vi "Response.vi"(8 "error in (no error)":errorcluster, 11 "Node Ptr":T2 format="%.0x") -> (0 "error out":errorcluster)   [LabVIEW 2018, in "Instrument Addon System Explorer.lvlib"]
uses:
  Instrument Addon System Explorer.lvlib
  <vilib>/NI Veristand/Custom Device API/Custom Device Item Ref.ctl
  Addon Shared/Types/Response Wait Type.ctl
  NationalInstruments.VeriStand.SystemStorageUI
  Addon Shared/Types/FG Control.ctl
  NationalInstruments.VeriStand.SystemStorage
  Addon Shared/SubVIs/Constants.vi
  <vilib>/NI Veristand/Custom Device API/NI VeriStand - Get Item Property.vi
  <vilib>/NI Veristand/Custom Device API/Get Item Property (String).vi
  <vilib>/NI Veristand/Custom Device API/Get Item Property (String Array).vi
  <vilib>/NI Veristand/Custom Device API/Get Item Property (Double).vi
  <vilib>/NI Veristand/Custom Device API/Get Item Property (U32).vi
  <vilib>/NI Veristand/Custom Device API/Get Item Property (Boolean).vi
  <vilib>/NI Veristand/Custom Device API/NI VeriStand - Set Item Property.vi
  <vilib>/NI Veristand/Custom Device API/Set Item Property (String).vi
  <vilib>/NI Veristand/Custom Device API/Set Item Property (String Array).vi
  <vilib>/NI Veristand/Custom Device API/Set Item Property (Double).vi
  <vilib>/NI Veristand/Custom Device API/Set Item Property (U32).vi
  <vilib>/NI Veristand/Custom Device API/Set Item Property (Boolean).vi
  <vilib>/NI Veristand/Custom Device API/Custom Device API.lvlib
  Addon Shared/Instrument Addon Shared.lvlib
  <vilib>/NI Veristand/UI Controls/Single Node Browser/NI_VS UI Single Node Browser.lvlib
panel:
  in  "Type Value U32":u32=100 caption="Byte Count Value"
  in  "Channel":refnum<k24>(container) caption="Value"
  in  "Use Channel?":bool
  in  "Linkages":i32(listbox)
  in  "MetaData":string(combo) caption="Available Data Channels"
  in  "Response":string caption="Response Format ( Use [] to define a variable )"
  in  "Header 2":cluster{"Section Name":string}={"Section Name"="Response Message Settings"}
  in  "Wait Type":T1
  in  "Type Value DBL":dbl=100.0 caption="Byte Count Value" format="%#_p"
  in  "SHDocVw.IWebBrowser":refnum<k7>(container)
  in  "Header":cluster{"Section Name":string}={"Section Name"="Response Settings"}
  in  "Description":string
  out "Name":string
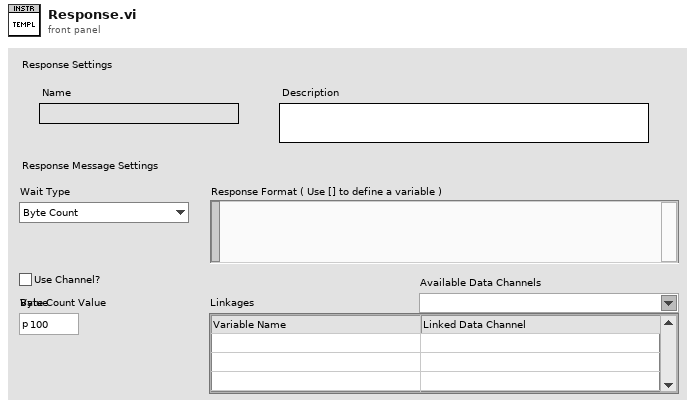
[diagram p1: front panel]
types:
  T1 = typedef "Instrument Addon Shared.lvlib/Response Wait Type.ctl" = enum16{"Byte Count", "Wait sec"}
  T2 = typedef "Custom Device API.lvlib/Custom Device Item Ref.ctl" = u64
  T3 = typedef "Instrument Addon Shared.lvlib/FG Control.ctl" = enum16{"Get", "Set"}
  T4 = typedef "Instrument Addon Shared.lvlib/Response Parameters.ctl" = cluster{"Response":string, "Linked Channels":T5[], "Type Value":dbl, "Wait Type":T1, "Use Channel":bool, "Channel Path":string}
  T5 = typedef "Instrument Addon Shared.lvlib/Linked Channel Cluster.ctl" = cluster{"Variable Name":string, "GUID":string}
  T6 = typedef "Custom Device API.lvlib/Custom Device Item Info.ctl" = cluster{"Name":string, "Is Channel":bool, "GUID":string, "Is Waveform":bool}
  T7 = typedef "Custom Device API.lvlib/Custom Device Commands.ctl" = enum16{"Default", "Item renamed", "Shutdown", "Dynamic button pressed"}
  T8 = typedef "NI_VS UI Single Node Browser.lvlib/Node Ref.ctl" = refnum<k24>
  T9 = typedef "Custom Device API.lvlib/Custom Device Pointer.ctl" = refnum<k24>
  T10 = typedef "LVComboBoxStrsAndValuesArrayTypeDef.ctl" = cluster{"String":string, "Value":string}[]
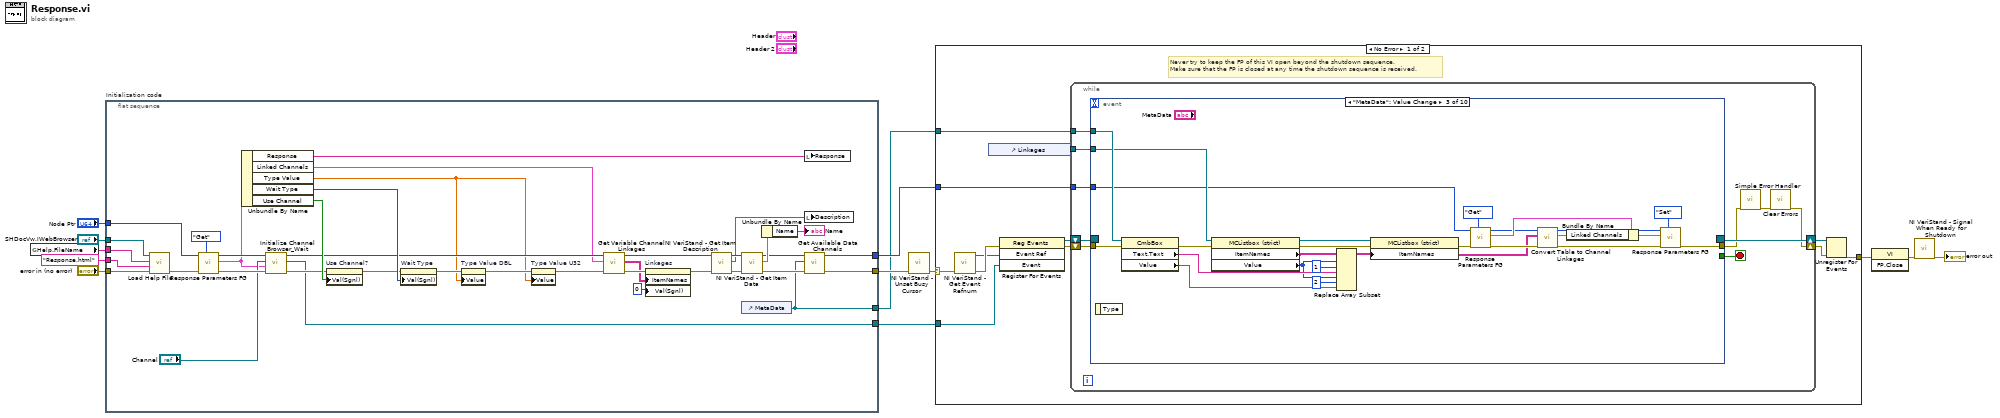
[diagram p0: block diagram]
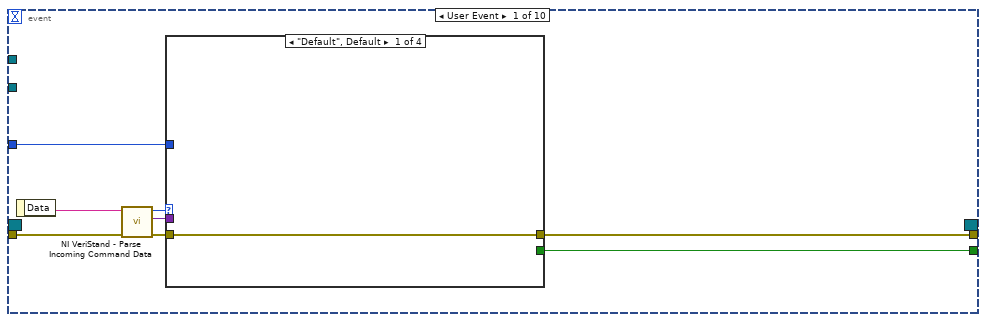
[diagram p2: hidden frame]
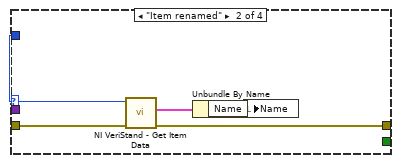
[diagram p3: hidden frame]
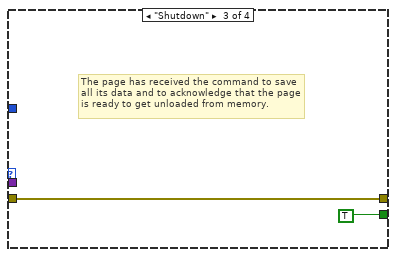
[diagram p4: hidden frame]
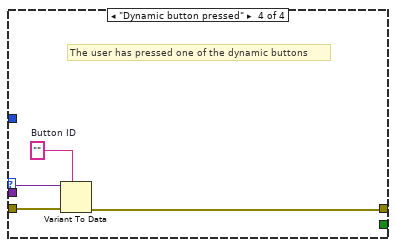
[diagram p5: hidden frame]
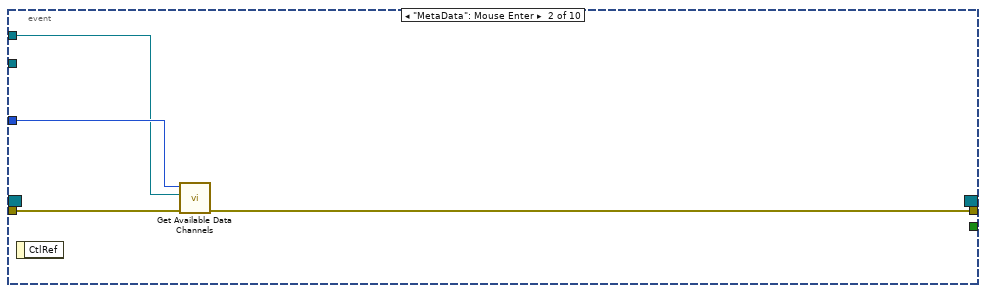
[diagram p6: hidden frame]
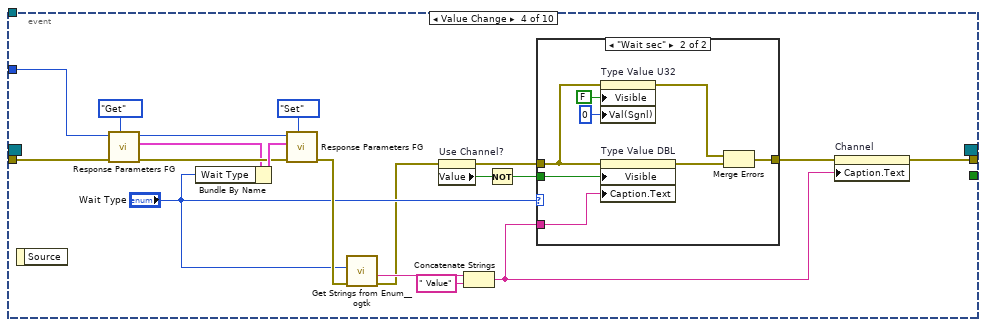
[diagram p7: hidden frame]
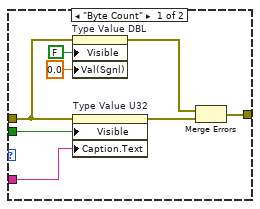
[diagram p8: hidden frame]
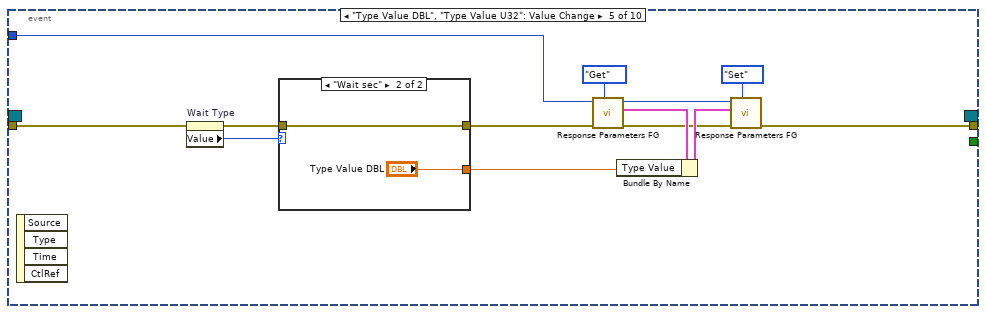
[diagram p9: hidden frame]
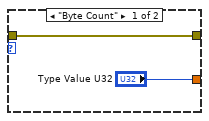
[diagram p10: hidden frame]
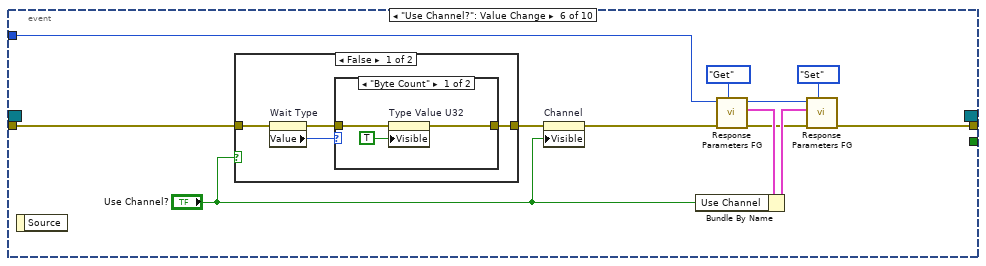
[diagram p11: hidden frame]
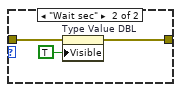
[diagram p12: hidden frame]
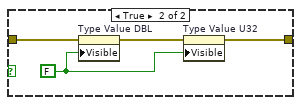
[diagram p13: hidden frame]
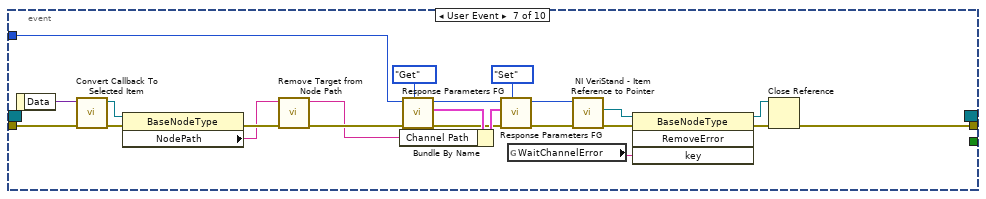
[diagram p14: hidden frame]
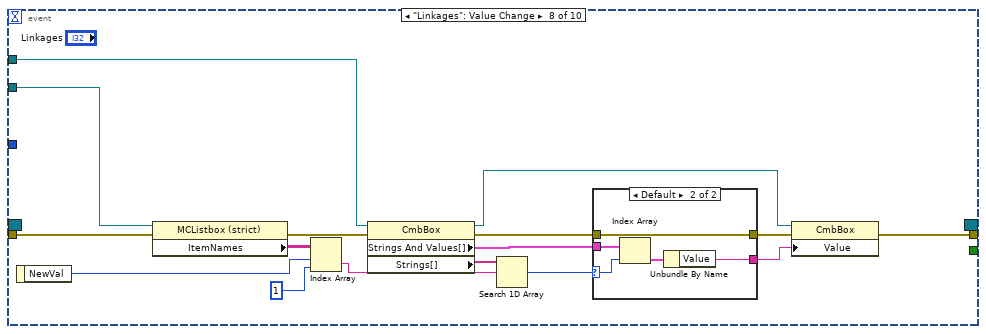
[diagram p15: hidden frame]
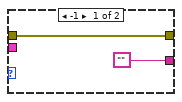
[diagram p16: hidden frame]
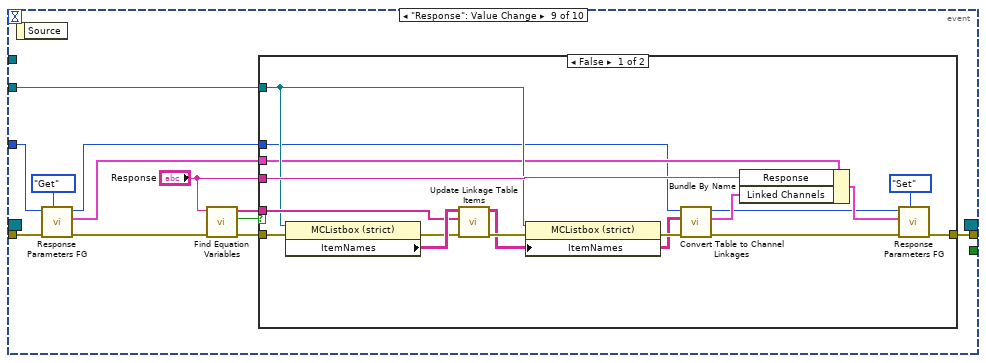
[diagram p17: hidden frame]
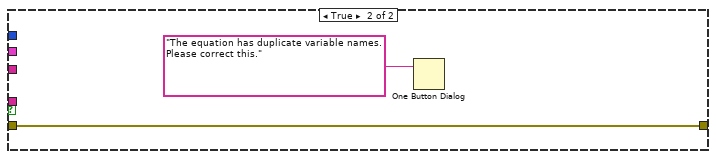
[diagram p18: hidden frame]
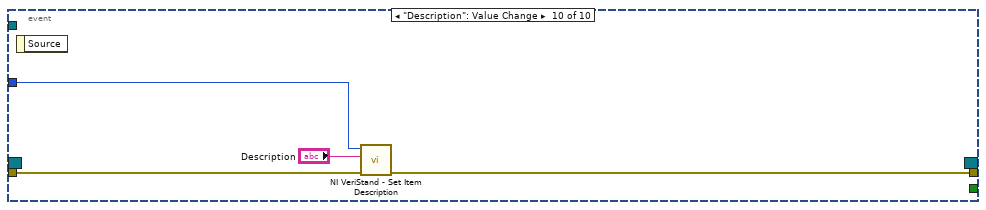
[diagram p19: hidden frame]
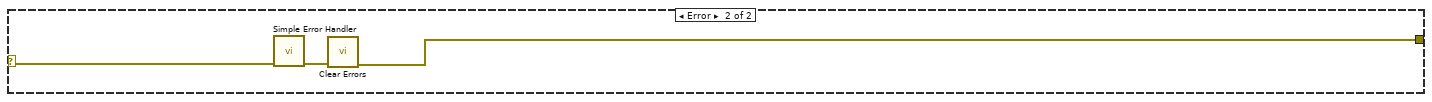
[diagram p20: hidden frame]
diagram:
  n1 = global read "Constants.vi" "Help.FileName"() -> (w1:string)
  n2 = flat-sequence "Initialization code" {
    tunnel: "error in (no error)" -> [w46]
    tunnel: "Node Ptr" -> [w41]
    tunnel: [w35] -> w9
    tunnel: [w33] -> w6
    tunnel: "SHDocVw.IWebBrowser" -> [w45]
    tunnel: "Response.html" ("HTML File") -> [w44]
    tunnel: w1 -> [w43]
    tunnel: [w32] -> w3
    tunnel: [w20] -> w2
    frame #0 {
      n3 = call "Load Help File.vi"("error in (no error)"=w46, "HTML File"=w44, "Main CHM File"=w43, "SHDocVw.IWebBrowser2"=w45) -> ("error out"=w42:errorcluster)  [unwired: 7 in]
      n4 = call "Response Parameters FG.vi"("Action"=FG_Control."Get", "error in (no error)"=w42, "Item Ref in"=w41) -> ("error out"=w24:errorcluster, "Response Parameters"=w17:T4, "Item Ref out"=w22:T2)  [unwired: 6 in]
      n5 = Unbundle By Name(w17) -> ("Response"=w37:string, "Linked Channels"=w18:T5[], "Type Value"=w14:dbl, "Wait Type"=w31:T1, "Use Channel"=w25:bool)
      n6 = call "Initialize Channel Browser_Wait.vi"("error in (no error)"=w24, "Reponse Parameters"=w17, ".NET Refnum in"="Channel", "Item Ref in"=w22) -> ("error out"=w23:errorcluster, "Event"=w20:refnum<user-event>, "Item Ref out"=w19:T2)  [unwired: 5 in]
      n7 = property on="Use Channel?" class="Bool (strict)"(error in=w23, "Val(Sgnl)"=w25) -> (error out=w26:errorcluster)  [unwired: 1 in, 1 out]
      n8 = property on="Wait Type" class="Enum (strict)"(error in=w26, "Val(Sgnl)"=w31) -> (error out=w27:errorcluster)  [unwired: 1 in, 1 out]
      n9 = property on="Type Value DBL" class="DigNum (strict)"(error in=w27, "Value"=w14) -> (error out=w16:errorcluster)  [unwired: 1 in, 1 out]
      n10 = property on="Type Value U32" class="DigNum (strict)"(error in=w16, "Value"=w14) -> (error out=w15:errorcluster)  [unwired: 1 in, 1 out]
      n11 = call "Get Variable Channel Linkages.vi"("error in (no error)"=w15, "Linked Channels"=w18, "Item Ref in"=w19) -> ("error out"=w30:errorcluster, "Array"=w28:string[][], "Item Ref out"=w29:T2)  [unwired: 6 in]
      n12 = property on="Linkages" class="MCListbox (strict)"(error in=w30, "ItemNames"=w28, "Val(Sgnl)"=0 ("Value (Signaling)")) -> (error out=w38:errorcluster)  [unwired: 1 in, 1 out]
      n13 = call <vilib>:"NI VeriStand - Get Item Description.vi"("error in (no error)"=w38, "Item Ref in"=w29) -> ("error out"=w49:errorcluster, "Description"=w50:string, "Item Ref out"=w51:T2)  [unwired: 7 out]
      n14 = control-ref of="MetaData"() -> (w32:refnum<vi>)
      n15 = call <vilib>:"NI VeriStand - Get Item Data.vi"("error in (no error)"=w49, "Item Ref in"=w51) -> ("error out"=w36:errorcluster, "Item Info"=w48:T6, "Item Ref out"=w34:T2)  [unwired: 7 out]
      n16 = Unbundle By Name(w48) -> ("Name"=→"Name":string)
      n17 = local write "Response"(w37) -> ()
      n18 = local write "Description"(w50) -> ()
      n19 = call "Get Available Data Channels.vi"("error in (no error)"=w36, "MetaData"=w32, "Item Ref in"=w34) -> ("error out"=w35:errorcluster, "Item Ref out"=w33:T2)  [unwired: 7 in]
    }
  }
  n20 = call <vilib>:"NI VeriStand - Unset Busy Cursor.vi"("error in (no error)"=w9) -> ("error out"=w8:errorcluster)  [unwired: 10 out]
  n21 = case shown="No Error" w8 {
    selector: w8 -> [w55 w284]
    tunnel: [w60 w282] -> w13
    tunnel: w6 -> [w56 _]
    tunnel: w3 -> [w53 _]
    tunnel: w2 -> [w52 _]
    frame No Error {
      # "Never try to keep the FP of this VI open beyond the shutdown sequence.\nMake sure that the FP is closed at any time the shutdown sequence is received."
      n22 = call <vilib>:"NI VeriStand - Get Event Refnum.vi"("error in (no error)"=w55) -> ("error out"=w63:errorcluster, "Event Ref"=w59:refnum<user-event>)  [unwired: 9 out]
      n23 = control-ref of="Linkages"() -> (w54:refnum<vi>)
      n24 = register-events(error in=w63, w59, w52) -> (reference out=w57:refnum<event-registration>, error out=w58:errorcluster)  [unwired: 1 in]
      n25 = while {
        tunnel: w56 -> [w69]
        shift-right: [w66] -> w61
        shift-left: w58 -> [w72]
        shift-right: [w73] -> w62
        shift-left: w57 -> [w71]
        tunnel: w54 -> [w64]
        tunnel: w53 -> [w65]
        stop <- w70 stop-if-true
        n26 = event shown="[2] \"MetaData\": Value Change" {
          selector: w71 -> [_ _ _ _ _ _ _ _ _ _]
          dyn-events: [_ _ _ _ _ _ _ _ _ _] -> w73
          timeout: _ -> [_ _ _ _ _ _ _ _ _ _]
          tunnel: w72 -> [w81 w97 w107 w136 w160 w177 w221 w228 w252 w280]
          tunnel: [w77 _ _ _ _ _ _ _ _ _] -> w70
          tunnel: [w76 w94 w103 w130 w162 w179 w203 w224 w255 w279] -> w68
          tunnel: w69 -> [w75 w96 w104 w137 w165 w178 w213 _ w250 w281]
          tunnel: w65 -> [_ w95 w106 _ _ _ _ w227 _ _]
          tunnel: w64 -> [_ _ w105 _ _ _ _ w226 w254 _]
          event User Event {
            n27 = event-data() -> ("Data"=w80:string)  [unwired: 1 out]
            n28 = call <vilib>:"NI VeriStand - Parse Incoming Command Data.vi"("error in (no error)"=w81, "Incoming data"=w80) -> ("error out"=w79:errorcluster, "Outgoing data"=w74:variant, "Action"=w78:T7)  [unwired: 7 out]
            n29 = case shown="\"Default\", Default" w78 {
              tunnel: w79 -> [w82 w87 w88 w93]
              tunnel: [_ _ TRUE _] -> w77
              tunnel: [w82 w84 w88 w90] -> w76
              tunnel: w75 -> [_ w86 _ _]
              tunnel: w74 -> [_ _ _ w92]
              frame "Default", Default {
              }
              frame "Item renamed" {
                n30 = call <vilib>:"NI VeriStand - Get Item Data.vi"("error in (no error)"=w87, "Item Ref in"=w86) -> ("error out"=w84:errorcluster, "Item Info"=w85:T6)  [unwired: 8 out]
                n31 = Unbundle By Name(w85) -> ("Name"=w83:string)
                n32 = local write "Name"(w83) -> ()
              }
              frame "Shutdown" {
                # "The page has received the command to save all its data and to acknowledge that the page is ready to get unloaded from memory."
              }
              frame "Dynamic button pressed" {
                w91 = ""  # Button ID
                # "The user has pressed one of the dynamic buttons"
                n33 = Variant To Data(error in=w93, type=w91, Variant=w92) -> (error out=w90:errorcluster)  [unwired: 1 out]
              }
            }
          }
          event "MetaData": Mouse Enter {
            n34 = event-data() -> ()  [unwired: 2 out]
            n35 = call "Get Available Data Channels.vi"("error in (no error)"=w97, "MetaData"=w95, "Item Ref in"=w96) -> ("error out"=w94:errorcluster)  [unwired: 7 in, 1 out]
          }
          event "MetaData": Value Change {
            n36 = event-data() -> ()  [unwired: 2 out]
            n37 = property class="CmbBox"(reference=w106, error in=w107) -> (error out=w110:errorcluster, "Text.Text"=w109:string, "Value"=w102:string)  [unwired: 1 out]
            n38 = property class="MCListbox (strict)"(reference=w105, error in=w110) -> (reference out=w120:refnum<vi>, error out=w119:errorcluster, "ItemNames"=w122:string[][], "Value"=w108:i32)
            n39 = Replace Array Subset(array=w122, new element #1=w109, index (row) #1=w108, index (col) #1=1 ("disabled index (col)"), new element #2=w102, index (row) #2=w108, index (col) #2=2 ("disabled index (col)")) -> (w101:string[][])
            n40 = property class="MCListbox (strict)"(reference=w120, error in=w119, "ItemNames"=w101) -> (error out=w114:errorcluster)  [unwired: 1 out]
            n41 = call "Response Parameters FG.vi"("Action"=FG_Control."Get", "error in (no error)"=w114, "Item Ref in"=w104) -> ("error out"=w113:errorcluster, "Response Parameters"=w112:T4, "Item Ref out"=w99:T2)  [unwired: 6 in]
            n42 = call "Convert Table to Channel Linkages.vi"("error in (no error)"=w113, "Item Names"=w101, "Item Ref in"=w99) -> ("error out"=w117:errorcluster, "Linkages"=w100:T5[], "Item Ref out"=w98:T2)  [unwired: 6 in]
            n43 = Bundle By Name(cluster=w112, "Linked Channels"=w100) -> (w116:T4)
            n44 = call "Response Parameters FG.vi"("Action"=FG_Control."Set", "error in (no error)"=w117, "Reponse Parameters"=w116, "Item Ref in"=w98) -> ("error out"=w103:errorcluster)  [unwired: 5 in, 2 out]
          }
          event Value Change {
            n45 = event-data() -> ()  [unwired: 2 out]
            n46 = call "Response Parameters FG.vi"("Action"=FG_Control."Get", "error in (no error)"=w136, "Item Ref in"=w137) -> ("error out"=w135:errorcluster, "Response Parameters"=w128:T4, "Item Ref out"=w138:T2)  [unwired: 6 in]
            n47 = Bundle By Name(cluster=w128, "Wait Type"="Wait Type") -> (w140:T4)
            n48 = call "Response Parameters FG.vi"("Action"=FG_Control."Set", "error in (no error)"=w135, "Reponse Parameters"=w140, "Item Ref in"=w138) -> ("error out"=w133:errorcluster)  [unwired: 5 in, 2 out]
            n49 = call <userlib>:"Get Strings from Enum__ogtk.vi"("error in (no error)"=w133, "Enum"="Wait Type") -> ("error out"=w126:errorcluster, "String Value"=w134:string)  [unwired: 6 in, 2 out]
            n50 = property on="Use Channel?" class="Bool (strict)"(error in=w126) -> (error out=w125:errorcluster, "Value"=w124:bool)  [unwired: 1 in, 1 out]
            n51 = Concatenate Strings(w134, " Value" ("string")) -> (w127:string)
            n52 = Not(x=w124) -> (.not. x?=w123:bool)
            n53 = case shown="\"Wait sec\"" "Wait Type" {
              tunnel: w125 -> [w147 w155]
              tunnel: [w146 w154] -> w131
              tunnel: w127 -> [w149 w157]
              tunnel: w123 -> [w142 w151]
              frame "Byte Count" {
                n54 = property on="Type Value DBL" class="DigNum (strict)"(error in=w147, "Visible"=FALSE, "Val(Sgnl)"=0.0 ("Value (Signaling)")) -> (error out=w145:errorcluster)  [unwired: 1 in, 1 out]
                n55 = property on="Type Value U32" class="DigNum (strict)"(error in=w147, "Visible"=w142, "Caption.Text"=w149) -> (error out=w148:errorcluster)  [unwired: 1 in, 1 out]
                n56 = Merge Errors(w145, w148) -> (w146:errorcluster)
              }
              frame "Wait sec" {
                n57 = property on="Type Value U32" class="DigNum (strict)"(error in=w155, "Visible"=FALSE, "Val(Sgnl)"=u32 0 ("Value (Signaling)")) -> (error out=w153:errorcluster)  [unwired: 1 in, 1 out]
                n58 = property on="Type Value DBL" class="DigNum (strict)"(error in=w155, "Visible"=w151, "Caption.Text"=w157) -> (error out=w156:errorcluster)  [unwired: 1 in, 1 out]
                n59 = Merge Errors(w153, w156) -> (w154:errorcluster)
              }
            }
            n60 = property on="Channel" class="AXCont"(error in=w131, "Caption.Text"=w127) -> (error out=w130:errorcluster)  [unwired: 1 in, 1 out]
          }
          event "Type Value DBL", "Type Value U32": Value Change {
            n61 = event-data() -> ()  [unwired: 5 out]
            n62 = property on="Wait Type" class="Enum (strict)"(error in=w160) -> (error out=w158:errorcluster, "Value"=w161:T1)  [unwired: 1 in, 1 out]
            n63 = case shown="\"Wait sec\"" w161 {
              tunnel: ["Type Value U32" "Type Value DBL"] -> w163
              tunnel: [w171 w173] -> w159
              tunnel: w158 -> [w171 w173]
              frame "Byte Count" {
              }
              frame "Wait sec" {
              }
            }
            n64 = call "Response Parameters FG.vi"("Action"=FG_Control."Get", "error in (no error)"=w159, "Item Ref in"=w165) -> ("error out"=w164:errorcluster, "Response Parameters"=w167:T4, "Item Ref out"=w166:T2)  [unwired: 6 in]
            n65 = Bundle By Name(cluster=w167, "Type Value"=w163) -> (w169:T4)
            n66 = call "Response Parameters FG.vi"("Action"=FG_Control."Set", "error in (no error)"=w164, "Reponse Parameters"=w169, "Item Ref in"=w166) -> ("error out"=w162:errorcluster)  [unwired: 5 in, 2 out]
          }
          event "Use Channel?": Value Change {
            n67 = event-data() -> ()  [unwired: 2 out]
            n68 = case shown="False" "Use Channel?" {
              tunnel: w177 -> [w190 w200]
              tunnel: [w187 w198] -> w176
              frame False {
                n69 = property on="Wait Type" class="Enum (strict)"(error in=w190) -> (error out=w188:errorcluster, "Value"=w189:T1)  [unwired: 1 in, 1 out]
                n70 = case shown="\"Byte Count\"" w189 {
                  tunnel: w188 -> [w193 w196]
                  tunnel: [w192 w195] -> w187
                  frame "Byte Count" {
                    n71 = property on="Type Value U32" class="DigNum (strict)"(error in=w193, "Visible"=TRUE) -> (error out=w192:errorcluster)  [unwired: 1 in, 1 out]
                  }
                  frame "Wait sec" {
                    n72 = property on="Type Value DBL" class="DigNum (strict)"(error in=w196, "Visible"=TRUE) -> (error out=w195:errorcluster)  [unwired: 1 in, 1 out]
                  }
                }
              }
              frame True {
                w197 = FALSE ("Visible")
                n73 = property on="Type Value DBL" class="DigNum (strict)"(error in=w200, "Visible"=w197) -> (error out=w199:errorcluster)  [unwired: 1 in, 1 out]
                n74 = property on="Type Value U32" class="DigNum (strict)"(error in=w199, "Visible"=w197) -> (error out=w198:errorcluster)  [unwired: 1 in, 1 out]
              }
            }
            n75 = property on="Channel" class="AXCont"(error in=w176, "Visible"="Use Channel?") -> (error out=w180:errorcluster)  [unwired: 1 in, 1 out]
            n76 = call "Response Parameters FG.vi"("Action"=FG_Control."Get", "error in (no error)"=w180, "Item Ref in"=w178) -> ("error out"=w181:errorcluster, "Response Parameters"=w183:T4, "Item Ref out"=w182:T2)  [unwired: 6 in]
            n77 = Bundle By Name(cluster=w183, "Use Channel"="Use Channel?") -> (w185:T4)
            n78 = call "Response Parameters FG.vi"("Action"=FG_Control."Set", "error in (no error)"=w181, "Reponse Parameters"=w185, "Item Ref in"=w182) -> ("error out"=w179:errorcluster)  [unwired: 5 in, 2 out]
          }
          event User Event {
            n79 = event-data() -> ("Data"=w220:variant)  [unwired: 1 out]
            n80 = call <vilib>:"Convert Callback To Selected Item.vi"("error in"=w221, "Data"=w220) -> ("error out"=w222:errorcluster, "Selected Item"=w223:T8)  [unwired: 8 in]
            n81 = property class="BaseNodeType"(reference=w223, error in=w222) -> (error out=w212:errorcluster, "NodePath"=w211:string)  [unwired: 1 out]
            n82 = call "Remove Target from Node Path.vi"("error in (no error)"=w212, "NodePath"=w211) -> ("error out"=w210:errorcluster, "PathArrayToString"=w209:string)  [unwired: 8 in]
            n83 = call "Response Parameters FG.vi"("Action"=FG_Control."Get", "error in (no error)"=w210, "Item Ref in"=w213) -> ("error out"=w214:errorcluster, "Response Parameters"=w216:T4, "Item Ref out"=w215:T2)  [unwired: 6 in]
            n84 = Bundle By Name(cluster=w216, "Channel Path"=w209) -> (w218:T4)
            n85 = call "Response Parameters FG.vi"("Action"=FG_Control."Set", "error in (no error)"=w214, "Reponse Parameters"=w218, "Item Ref in"=w215) -> ("error out"=w204:errorcluster, "Item Ref out"=w202:T2)  [unwired: 5 in, 1 out]
            n86 = global read "Constants.vi" "WaitChannelError"() -> (w201:string)
            n87 = call <vilib>:"NI VeriStand - Item Reference to Pointer.vi"("error in (no error)"=w204, "Item Ref in"=w202) -> ("error out"=w206:errorcluster, "Node Pointer"=w205:T9)  [unwired: 6 in, 2 out]
            n88 = invoke class="BaseNodeType" method="RemoveError"(reference=w205, error in=w206, "key"=w201) -> (reference out=w208:T9, error out=w207:errorcluster)  [unwired: 1 in, 2 out]
            n89 = Close Reference(reference=w208, error in (no error)=w207) -> (error out=w203:errorcluster)
          }
          event "Linkages": Value Change {
            n90 = event-data() -> ("NewVal"=w225:i32)  [unwired: 1 out]
            n91 = property class="MCListbox (strict)"(reference=w226, error in=w228) -> (error out=w237:errorcluster, "ItemNames"=w239:string[][])  [unwired: 1 out]
            n92 = Index Array(array=w239, index (row)=w225, index (col)=1 ("disabled index (col)")) -> (element=w236:string)
            n93 = property class="CmbBox"(reference=w227, error in=w237) -> (reference out=w232:refnum<vi>, error out=w230:errorcluster, "Strings And Values[]"=w235:T10, "Strings[]"=w229:string[])
            n94 = Search 1D Array(1D array=w229, element=w236) -> (index of element=w233:i32)  [unwired: 1 in]
            n95 = case shown="Default" w233 {
              selector: w233 -> [_ w244]
              tunnel: w235 -> [_ w246]
              tunnel: ["" w242] -> w234
              tunnel: [w241 w243] -> w231
              tunnel: w230 -> [w241 w243]
              frame -1 {
              }
              frame Default {
                n96 = Index Array(array=w246, index=w244) -> (element=w245:cluster{"String":string, "Value":string})
                n97 = Unbundle By Name(w245) -> ("Value"=w242:string)
              }
            }
            n98 = property class="CmbBox"(reference=w232, error in=w231, "Value"=w234) -> (error out=w224:errorcluster)  [unwired: 1 out]
          }
          event "Response": Value Change {
            n99 = event-data() -> ()  [unwired: 2 out]
            n100 = call "Response Parameters FG.vi"("Action"=FG_Control."Get", "error in (no error)"=w252, "Item Ref in"=w250) -> ("error out"=w251:errorcluster, "Response Parameters"=w248:T4, "Item Ref out"=w249:T2)  [unwired: 6 in]
            n101 = call "Find Equation Variables.vi"("error in (no error)"=w251, "Command"="Response") -> ("error out"=w258:errorcluster, "Duplicate?"=w247:bool, "Variables"=w257:string[])  [unwired: 7 in]
            n102 = case shown="False" w247 {
              tunnel: w258 -> [w269 w277]
              tunnel: w257 -> [w268 _]
              tunnel: "Response" -> [w267 _]
              tunnel: [w266 w277] -> w255
              tunnel: w254 -> [w265 _]
              tunnel: w249 -> [w260 _]
              tunnel: w248 -> [w264 _]
              frame False {
                n103 = property class="MCListbox (strict)"(reference=w265, error in=w269) -> (error out=w270:errorcluster, "ItemNames"=w271:string[][])  [unwired: 1 out]
                n104 = call "Update Linkage Table Items.vi"("error in (no error)"=w270, "Variables"=w268, "Item Names"=w271) -> ("error out"=w272:errorcluster, "Item Names"=w262:string[][])  [unwired: 7 in]
                n105 = property class="MCListbox (strict)"(reference=w265, error in=w272, "ItemNames"=w262) -> (error out=w274:errorcluster)  [unwired: 1 out]
                n106 = call "Convert Table to Channel Linkages.vi"("error in (no error)"=w274, "Item Names"=w262, "Item Ref in"=w260) -> ("error out"=w275:errorcluster, "Linkages"=w261:T5[], "Item Ref out"=w259:T2)  [unwired: 6 in]
                n107 = Bundle By Name(cluster=w264, "Response"=w267, "Linked Channels"=w261) -> (w263:T4)
                n108 = call "Response Parameters FG.vi"("Action"=FG_Control."Set", "error in (no error)"=w275, "Reponse Parameters"=w263, "Item Ref in"=w259) -> ("error out"=w266:errorcluster)  [unwired: 5 in, 2 out]
              }
              frame True {
                n109 = One Button Dialog(message="The equation has duplicate variable names.  Please correct this.") -> ()  [unwired: 1 in, 1 out]
              }
            }
          }
          event "Description": Value Change {
            n110 = event-data() -> ()  [unwired: 2 out]
            n111 = call <vilib>:"NI VeriStand - Set Item Description.vi"("error in (no error)"=w280, "Description"="Description", "Item Ref in"=w281) -> ("error out"=w279:errorcluster)  [unwired: 8 out]
          }
        }
        n112 = call <vilib>:"Simple Error Handler.vi"("error in (no error)"=w68) -> ("error out"=w67:errorcluster)  [unwired: 1 in, 7 out]
        n113 = call <vilib>:"Clear Errors.vi"("error in (no error)"=w67) -> ("error out"=w66:errorcluster)  [unwired: 1 in, 5 out]
      }
      n114 = Unregister For Events(event registration refnum=w62, error in=w61) -> (error out=w60:errorcluster)
    }
    frame Error {
      n115 = call <vilib>:"Simple Error Handler.vi"("error in (no error)"=w284) -> ("error out"=w283:errorcluster)  [unwired: 1 in, 7 out]
      n116 = call <vilib>:"Clear Errors.vi"("error in (no error)"=w283) -> ("error out"=w282:errorcluster)  [unwired: 1 in, 5 out]
    }
  }
  n117 = invoke class="VI" method="FP.Close"(error in=w13) -> (error out=w12:errorcluster)  [unwired: 2 in, 2 out]
  n118 = call <vilib>:"NI VeriStand - Signal When Ready for Shutdown.vi"("error in (no error)"=w12) -> ("error out"=→"error out":errorcluster)  [unwired: 10 out]
